vi "Rysowanie punktu.vi"(9 "Punkt na mapie":T2={"Położenie"={"Pixel x"=0, "Pixel y"=0}, "Kolor punktu"=0, "Rozmiar punktu"=2, "Nazwa punktu"=""}, 10 "Właściwości mapy":T1={"Przesunięcie mapy"={"X"=0, "Y"=0}, "Zoom"=1.0, "Długość piksela w metrach"=0.01}, 11 "Mapa terenu":picture) -> (3 "Mapa z wprowadzonym punktem":picture)   [LabVIEW 2012, in "Biblioteka moduł map v3.lvlib" / "Obsługa grafiki mapy.lvlib"]
doc: "Zadaniem pliku jest dorysowanie do aktualnej mapy terenu punktu o zadanych właściwościach (kolor, nazwa, rozmiar, położenie względem lewego górnego rogu mapy) z uwzględnieniem parametrów wgranej mapy (zoom mapy, przesunięcie mapy)."
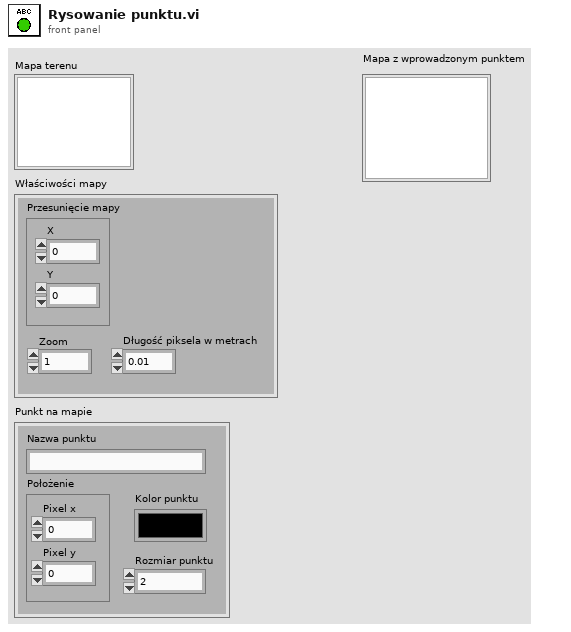
[diagram p1: front panel]
types:
  T1 = cluster{"Przesunięcie mapy":cluster{"X":i16, "Y":i16}, "Zoom":dbl, "Długość piksela w metrach":dbl}
  T2 = cluster{"Położenie":cluster{"Pixel x":i16, "Pixel y":i16}, "Kolor punktu":u32, "Rozmiar punktu":u32, "Nazwa punktu":string}
  T3 = cluster{"Width":u16, "Style":enum32{"Solid", "Dash", "Dot", "DashDot", "DashDotDot"}}
  T4 = cluster{"left":i16, "top":i16, "right":i16, "bottom":i16}
  T5 = enum16{"User-specified Font", "Application Font", "System Font", "Dialog Font"}
  T6 = cluster{"Font Name:":string, "Size":dbl, "Strikeout?":bool, "Italic?":bool, "Underline?":bool, "Outline?":bool, "Shadow?":bool, "Bold?":bool}
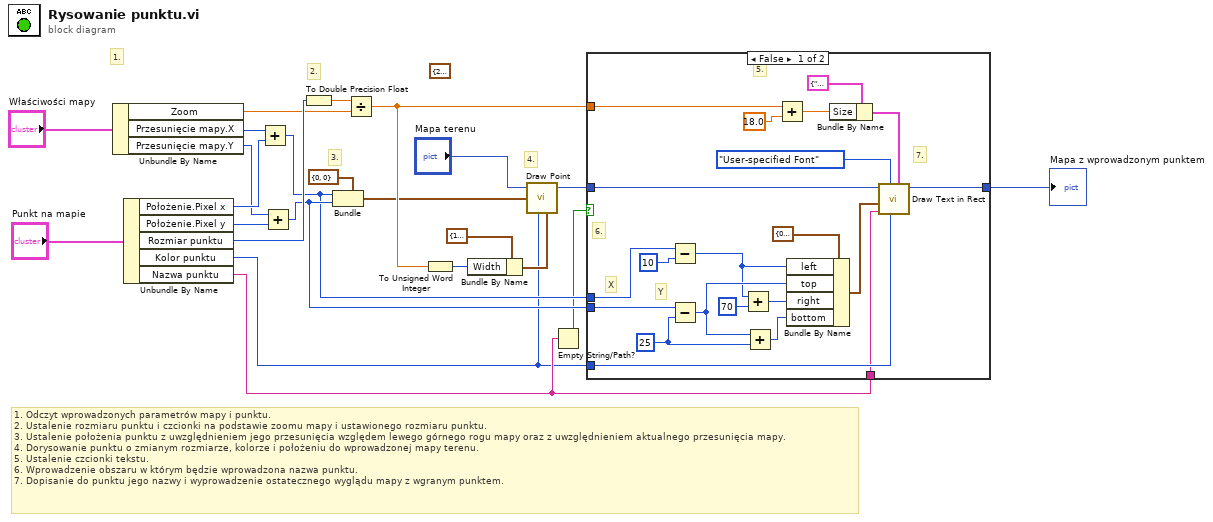
[diagram p0: block diagram]
diagram:
  (unwired) T3 {"Width"=2, "Style"=enum."Solid"} ("pen")
  # "1. Odczyt wprowadzonych parametrów mapy i punktu.\n2. Ustalenie rozmiaru punktu i czcionki na podstawie zoomu mapy i ustawionego rozmiaru punktu.\n3. Ustalenie położenia punktu z uwzględnieniem jego przesunięcia względem lewego górnego rogu mapy oraz z uwzględnieniem aktualnego przesunięcia mapy.\n4. Dorysowanie punktu o zmianym rozmiarze, kolorze i położeniu do wprowadzonej mapy terenu.\n5. Ustalenie czcionki tekstu.\n6. Wprowadzenie obszaru w którym będzie wprowadzona nazwa punktu.\n7. Dopisanie do punktu jego nazwy i wyprowadzenie ostatecznego wyglądu mapy z wgranym punktem."
  # "4."
  # "3."
  # "2."
  # "1."
  n1 = Unbundle By Name("Właściwości mapy") -> ("Zoom"=w18:dbl, "Przesunięcie mapy.X"=w17:i16, "Przesunięcie mapy.Y"=w11:i16)
  n2 = Unbundle By Name("Punkt na mapie") -> ("Położenie.Pixel x"=w15:i16, "Położenie.Pixel y"=w12:i16, "Rozmiar punktu"=w19:u32, "Kolor punktu"=w1:u32, "Nazwa punktu"=w8:string)
  n3 = Add(x=w17, y=w15) -> (x+y=w9:i16)
  n4 = Add(x=w11, y=w12) -> (x+y=w10:i16)
  n5 = To Double Precision Float(number=w19) -> (double precision float=w20:dbl)
  n6 = Bundle(cluster=cluster{"x":i16, "y":i16} {"x"=0, "y"=0} ("x+y"), "x"=w9, "y"=w10) -> (w4:cluster{"x":i16, "y":i16})
  n7 = Divide(x=w20, y=w18) -> (x/y=w13:dbl)
  n8 = To Unsigned Word Integer(number=w13) -> (unsigned 16bit integer=w14:u16)
  n9 = Bundle By Name(cluster=T3 {"Width"=1, "Style"=enum."Solid"} ("pen"), "Width"=w14) -> (w2:T3)
  n10 = call <vilib>:"Draw Point.vi"("picture"="Mapa terenu", "point(x,y)"=w4, "color(black)"=w1, "pen"=w2) -> ("new picture"=w6:picture)  [unwired: 5 in]
  n11 = Empty String/Path?(string/path=w8) -> (empty?=w7:bool)
  n12 = case shown="False" w7 {
    tunnel: [w44 w45] -> w23
    tunnel: w6 -> [w32 w45]
    tunnel: w1 -> [w31 _]
    tunnel: w13 -> [w27 _]
    tunnel: w10 -> [w26 _]
    tunnel: w9 -> [w25 _]
    tunnel: w8 -> [w24 _]
    frame False {
      w43 = i16 25 ("bottom")
      # "Y"
      # "X"
      # "7."
      # "6."
      # "5."
      n13 = Subtract(x=w25, y=i16 10) -> (x-y=w40:i16)
      n14 = Subtract(x=w26, y=w43) -> (x-y=w42:i16)
      n15 = Add(x=w40, y=i16 70 ("right")) -> (x+y=w34:i16)
      n16 = Add(x=w42, y=w43) -> (x+y=w35:i16)
      n17 = Add(x=w27, y=18.0) -> (x+y=w30:dbl)
      n18 = Bundle By Name(cluster=T4 {"left"=0, "top"=0, "right"=0, "bottom"=0} ("rect"), "left"=w40, "top"=w42, "right"=w34, "bottom"=w35) -> (w37:T4)
      n19 = Bundle By Name(cluster=T6 {"Font Name:"="Arial", "Size"=16.0, "Strikeout?"=FALSE, "Italic?"=FALSE, "Underline?"=FALSE, "Outline?"=FALSE, "Shadow?"=FALSE, "Bold?"=FALSE} ("[user-specified font]"), "Size"=w30) -> (w39:T6)
      n20 = call <vilib>:"Draw Text in Rect.vi"("[user-specified font]"=w39, "text color(black)"=w31, "desired font(Application)"=T5."User-specified Font", "text"=w24, "rect"=w37, "picture"=w32) -> ("new picture"=w44:picture)  [unwired: 5 in]
    }
    frame True {
    }
  }
  "Mapa z wprowadzonym punktem" <- w23
